vi "Check Connection.vi"(8 "error in (no error)":errorcluster, 11 "Potentiostat Galvanostat in":refnum<class "Potentiostat Galvanostat.lvclass">) -> (0 "error out":errorcluster, 2 "Connected?":bool, 3 "Potentiostat Galvanostat out":refnum<class "Potentiostat Galvanostat.lvclass">)   [LabVIEW 2018, in "Potentiostat Galvanostat.lvclass"]
uses:
  Potentiostat Galvanostat.lvclass
  Potentiostat Galvanostat.lvclass/Potentiostat Galvanostat.ctl
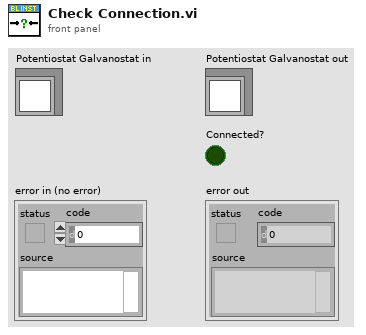
[diagram p1: front panel]
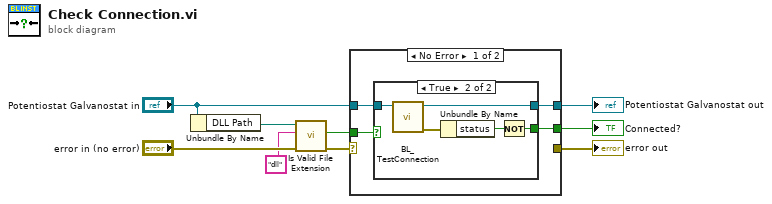
[diagram p0: block diagram]
diagram:
  n1 = Unbundle By Name("Potentiostat Galvanostat in") -> ("DLL Path"=w6:path)
  n2 = call "Is Valid File Extension.vi"("error in (no error)"="error in (no error)", "File extension"="dll", "Path"=w6) -> ("error out"=w2:errorcluster, "Is Valid File Extension?"=w3:bool)  [unwired: 6 in, 1 out]
  n3 = case shown="No Error" w2 {
    selector: w2 -> [_ w21]
    tunnel: [w13 w20] -> w9
    tunnel: [w12 _] -> w8
    tunnel: "Potentiostat Galvanostat in" -> [w11 w20]
    tunnel: w3 -> [w10 _]
    tunnel: [_ w21] -> w1
    frame No Error {
      n4 = case shown="True" w10 {
        tunnel: [w14 w19] -> w13
        tunnel: [_ w18] -> w12
        tunnel: w11 -> [w14 w15]
        frame False {
        }
        frame True {
          n5 = call "BL_TestConnection.vi"("Potentiostat Galvanostat in"=w15) -> ("error out"=w17:errorcluster, "Potentiostat Galvanostat out"=w19:refnum<class "Potentiostat Galvanostat.lvclass">)  [unwired: 9 in]
          n6 = Unbundle By Name(w17) -> ("status"=w16:bool)
          n7 = Not(x=w16) -> (.not. x?=w18:bool)
        }
      }
    }
    frame Error {
    }
  }
  "error out" <- w1
  "Potentiostat Galvanostat out" <- w9
  "Connected?" <- w8
